vi "[RT]Loop_Recieve.vi"(11 "myRIO_BefehlsQueue":refnum<queue>) -> ()   [LabVIEW 2018]
uses:
  TypeDef/CMD Cluster.ctl
  TypeDef/ControllerState.ctl
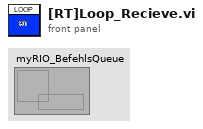
[diagram p1: front panel]
types:
  T1 = typedef "ControllerState.ctl" = enum16{"Idle", "Vorheizen", "Brühen", "Emergency-Stop"}
  T2 = typedef "CMD Cluster.ctl" = cluster{"timestamp":u32, "State Rqst":T1, "target-temp":dbl, "target-volume":dbl}
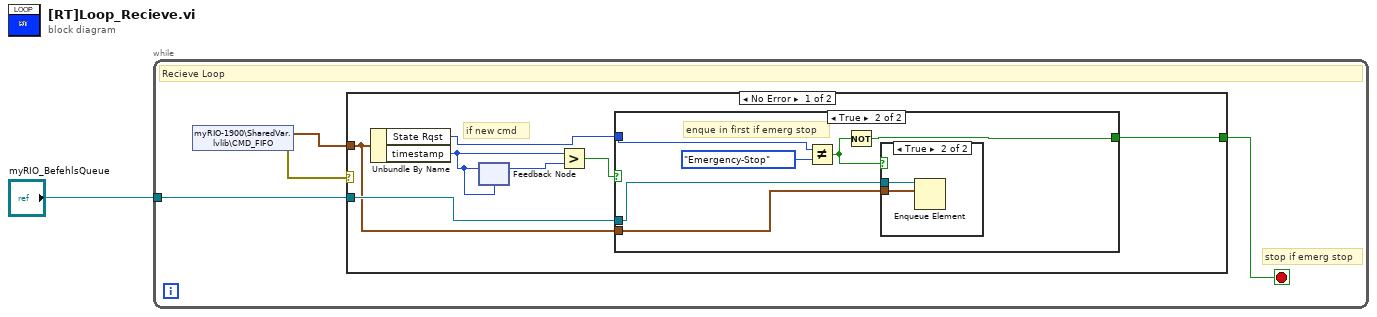
[diagram p0: block diagram]
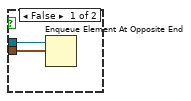
[diagram p3: hidden frame]
diagram:
  n1 = while {
    tunnel: "myRIO_BefehlsQueue" -> [w5]
    stop <- w2 stop-if-true
    # "stop if emerg stop"
    # "Recieve Loop"
    n2 = shared-variable "myRIO-1900\\SharedVar.lvlib\\CMD_FIFO"() -> (w4:T2, error out=w3:errorcluster)  [unwired: 1 in]
    n3 = case shown="No Error" w3 {
      tunnel: w5 -> [w10 _]
      tunnel: w4 -> [w9 _]
      tunnel: [w7 _] -> w2
      frame No Error {
        # "if new cmd"
        n4 = Unbundle By Name(w9) -> ("State Rqst"=w8:T1, "timestamp"=w6:u32)
        n5 = feedback #1(w6) -> (w12:u32)
        n6 = feedback-in #1(w6) -> ()
        n7 = Greater?(x=w6, y=w12) -> (0:w11:bool)
        n8 = case shown="True" w11 {
          tunnel: w10 -> [_ w18]
          tunnel: w9 -> [_ w17]
          tunnel: w8 -> [_ w16]
          tunnel: [_ w13] -> w7
          frame False {
          }
          frame True {
            # "enque in first if emerg stop"
            n9 = Not Equal?(x=w16, y=ControllerState."Emergency-Stop") -> (x != y?=w14:bool)
            n10 = Not(x=w14) -> (.not. x?=w13:bool)
            n11 = case shown="True" w14 {
              tunnel: w18 -> [w19 w22]
              tunnel: w17 -> [w20 w21]
              frame False {
                n12 = Enqueue Element At Opposite End(queue=w19, element=w20) -> ()  [unwired: 2 in, 3 out]
              }
              frame True {
                n13 = Enqueue Element(queue=w22, element=w21) -> ()  [unwired: 2 in, 3 out]
              }
            }
          }
        }
      }
      frame Error {
      }
    }
  }
